vi "NI tdms viewer.vi"() -> ()   [LabVIEW 2017, in "util.lvlib"]
uses:
  util.lvlib
panel:
  in  "file path":path caption="Dateipfad"
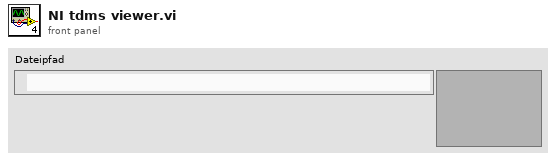
[diagram p1: front panel]
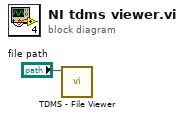
[diagram p0: block diagram]
diagram:
  n1 = call <vilib>:"TDMS - File Viewer.vi"("file path"="file path") -> ()  [unwired: 5 in, 2 out]
